vi "DataFinder List Indexed Properties.vi"(8 "error in (no error)":errorcluster, 10 "Type (tdm_file)":T1(ring), 11 "DataFinder (\"My DataFinder\")":string="My DataFinder") -> (0 "error out":errorcluster, 3 "Indexed Properties":T3(array[cluster]))   [LabVIEW 2011]
uses:
  DataFinder Indexed Property DataTypes.ctl
panel:
  out "Table Control":string[][](table)
  in  "SUSIQueryForm":refnum<k7>(container)
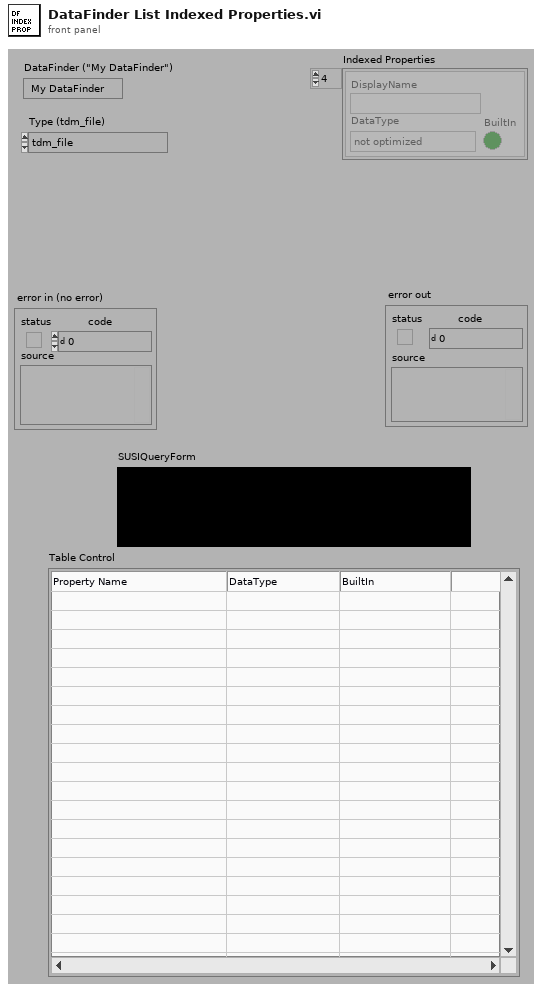
[diagram p1: front panel]
types:
  T1 = enum16{"tdm_file", "tdm_channelgroup", "tdm_channel"}
  T2 = typedef "DataFinder Indexed Property DataTypes.ctl" = enum32{"not optimized", "string", "double", "integer"}
  T3 = cluster{"DisplayName":string, "DataType":T2, "BuiltIn":bool}[]
  T4 = cluster{"DisplayName":string, "DataType":T2, bool}
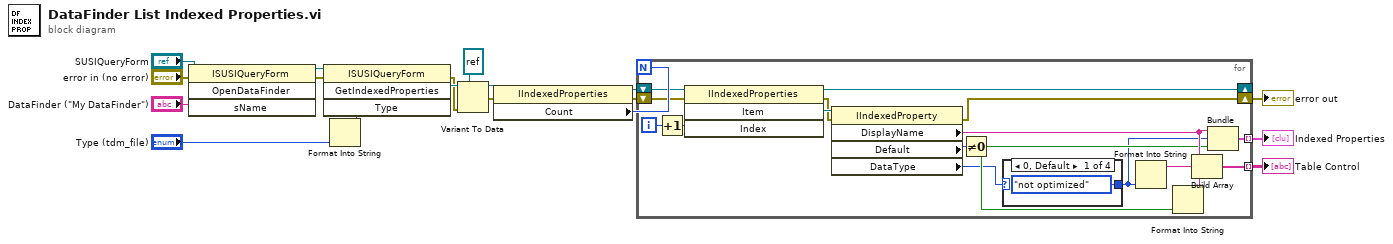
[diagram p0: block diagram]
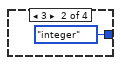
[diagram p2: hidden frame]
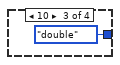
[diagram p3: hidden frame]
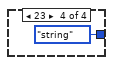
[diagram p4: hidden frame]
diagram:
  n1 = invoke class="ISUSIQueryForm" method="OpenDataFinder"(reference="SUSIQueryForm", error in="error in (no error)", "sName"="DataFinder (\"My DataFinder\")") -> (reference out=w5:refnum<k7>, error out=w2:errorcluster)  [unwired: 1 in, 2 out]
  n2 = Format Into String("Type (tdm_file)") -> (resulting string=w4:string)  [unwired: 3 in, 1 out]
  n3 = invoke class="ISUSIQueryForm" method="GetIndexedProperties"(reference=w5, error in=w2, "Type"=w4) -> (reference out=w3:refnum<k7>, error out=w1:errorcluster)  [unwired: 1 in, 2 out]
  n4 = Variant To Data(error in=w1, type=refnum<k7> refnum ("reference"), Variant=w3) -> (data=w7:refnum<k7>, error out=w6:errorcluster)
  n5 = property class="IIndexedProperties"(reference=w7, error in=w6) -> (reference out=w16:refnum<k7>, error out=w15:errorcluster, "Count"=w17:i32)
  n6 = for {
    N: w17 -> [_]
    shift-right: [w34] -> _
    shift-left: w16 -> [w35]
    shift-right: [w28] -> w10
    shift-left: w15 -> [w33]
    tunnel: [w27] -> w11 mode=indexing
    tunnel: [w24] -> w9 mode=indexing
    i -> [w31]
    n7 = Increment(x=w31) -> (x+1=w30:i32)
    n8 = invoke class="IIndexedProperties" method="Item"(reference=w35, error in=w33, "Index"=w30) -> (reference out=w34:refnum<k7>, error out=w29:errorcluster, "Item"=w32:refnum<k7>)  [unwired: 1 in, 1 out]
    n9 = property class="IIndexedProperty"(reference=w32, error in=w29) -> (error out=w28:errorcluster, "DisplayName"=w23:string, "Default"=w22:i32, "DataType"=w19:i32)  [unwired: 1 out]
    n10 = Not Equal To 0?(x=w22) -> (x != 0?=w21:bool)
    n11 = case shown="0, Default" w19 {
      tunnel: [DataFinder_Indexed_Property_DataTypes."not optimized" ("DataType") DataFinder_Indexed_Property_DataTypes."integer" ("DataType") DataFinder_Indexed_Property_DataTypes."double" ("DataType") DataFinder_Indexed_Property_DataTypes."string" ("DataType")] -> w20
      frame 0, Default {
      }
      frame 3 {
      }
      frame 10 {
      }
      frame 23 {
      }
    }
    n12 = Format Into String(w20) -> (resulting string=w26:string)  [unwired: 3 in, 1 out]
    n13 = Format Into String(w21) -> (resulting string=w25:string)  [unwired: 3 in, 1 out]
    n14 = Build Array(w23, w26, w25) -> (w24:string[])
    n15 = Bundle("DisplayName"=w23, "DataType"=w20, w21) -> (w27:T4)  [unwired: 1 out]
  }
  "error out" <- w10
  "Indexed Properties" <- w11
  "Table Control" <- w9
